vi "Read Container.vi"(8 "error in (no error)":errorcluster, 11 "Syringe Line in":refnum<class "Syringe Line.lvclass">) -> (0 "error out":errorcluster, 1 "Sample":refnum<class "Sample.lvclass">, 2 "Container":T1, 3 "Syringe Line out":refnum<class "Syringe Line.lvclass">)   [LabVIEW 2015, in "cRIO-Carbondioxide.lvlib" / "CO2-Actor.lvlib" / "Syringe Line.lvclass"]
uses:
  Syringe Line.lvclass
  Controls/Sample Container.ctl
  subs/Sample/Sample.lvclass
  Syringe Line.lvclass/Syringe Line.ctl
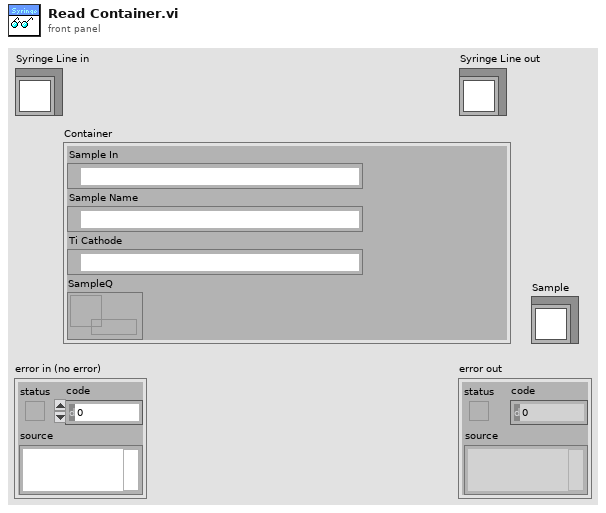
[diagram p1: front panel]
types:
  T1 = typedef "Sample Container.ctl" = cluster{"Sample In":refnum<k21>, "Sample Name":refnum<k21>, "Ti Cathode":refnum<k21>, "SampleQ":refnum<queue>}
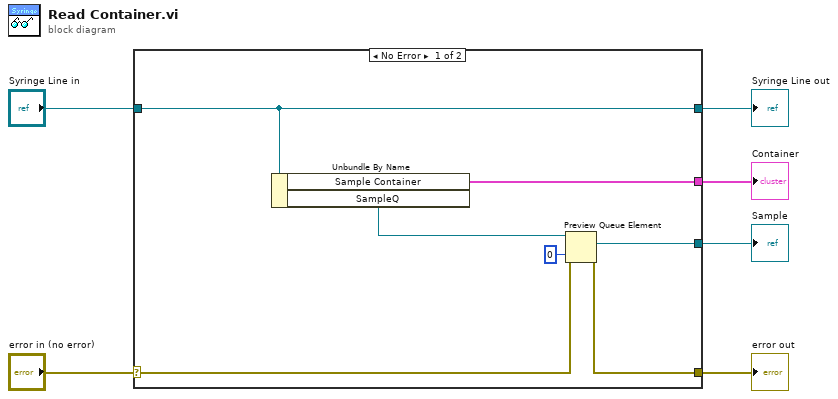
[diagram p0: block diagram]
diagram:
  n1 = case shown="No Error" "error in (no error)" {
    selector: "error in (no error)" -> [w9 w15]
    tunnel: [w8 w15] -> w5
    tunnel: [w13 w14] -> w3
    tunnel: "Syringe Line in" -> [w13 w14]
    tunnel: [w12 _] -> w2
    tunnel: [w10 _] -> w1
    frame No Error {
      n2 = Unbundle By Name(w13) -> ("Sample Container"=w12:T1, "SampleQ"=w7:refnum<queue>)
      n3 = Preview Queue Element(queue=w7, timeout in ms (-1)=0, error in (no error)=w9) -> (element=w10:refnum<class "Sample.lvclass">, error out=w8:errorcluster)  [unwired: 2 out]
    }
    frame Error {
    }
  }
  "error out" <- w5
  "Syringe Line out" <- w3
  "Sample" <- w1
  "Container" <- w2
